vi "mkGetROIs.vi"(10 "Camera settings":T1={"Gain [1-4]"=0.0, "Offset"=0, "Mode"=0, "ROIs"=[], "ROI Size"={"X"=0, "Y"=0}, "Number of buffers"=40, "Use hardware multiple-ROI?"=TRUE, "GenericCameraConfig"={"Framerate (Hz)"=60, "Exposure time (us)"=5000, "Image size"={"Width"=1280, "Height"=1024}, "Number of buffers"=30}}, 11 "IMAQ Refnum in":refnum<k11>) -> (2 "Camera settings (out)":T1={"Gain [1-4]"=0.0, "Offset"=0, "Mode"=0, "ROIs"=[], "ROI Size"={"X"=0, "Y"=0}, "Number of buffers"=40, "Use hardware multiple-ROI?"=TRUE, "GenericCameraConfig"={"Framerate (Hz)"=60, "Exposure time (us)"=5000, "Image size"={"Width"=1280, "Height"=1024}, "Number of buffers"=30}}, 3 "IMAQ Refnum out":refnum<k11>)   [LabVIEW 2011]
uses:
  CameraConfig.ctl
  Main/Camera/GenericCameraConfigType.ctl
panel:
  out "#ROI":i32
  # "us"
  # "us"
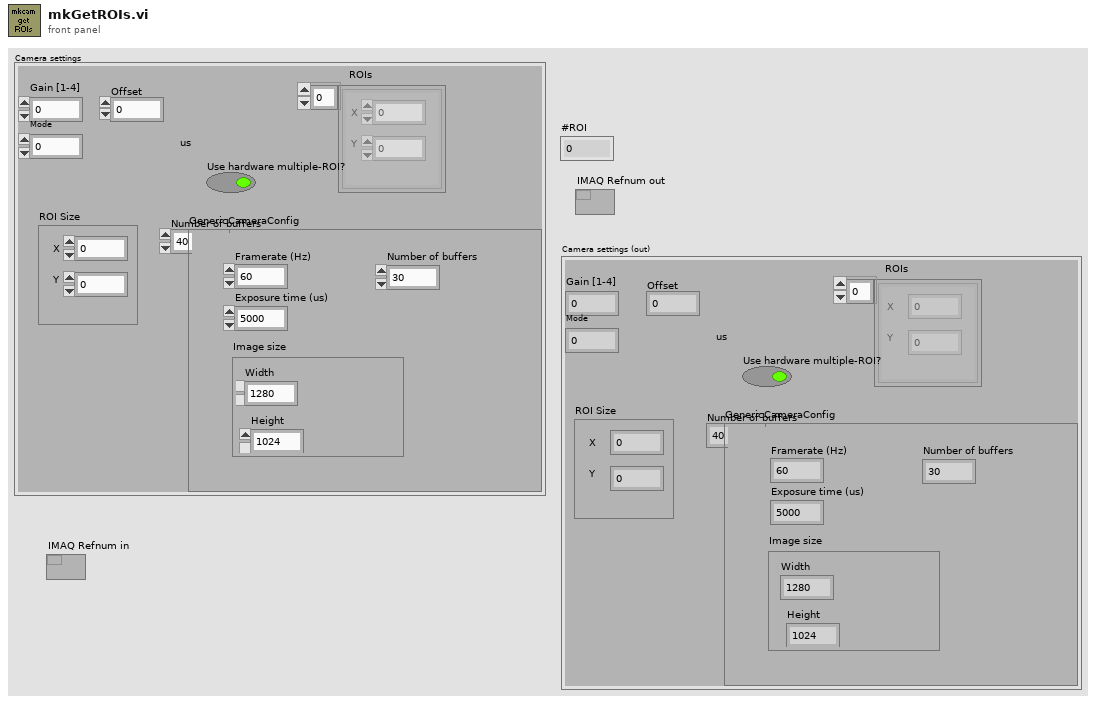
[diagram p1: front panel]
types:
  T1 = typedef "CameraConfig.ctl" = cluster{"Gain [1-4]":sgl, "Offset":i16, "Mode":i16, "ROIs":cluster{"X":i32, "Y":i32}[], "ROI Size":cluster{"X":i32, "Y":i32}, "Number of buffers":i32, "Use hardware multiple-ROI?":bool, "GenericCameraConfig":T2}
  T2 = typedef "GenericCameraConfigType.ctl" = cluster{"Framerate (Hz)":i32, "Exposure time (us)":i32, "Image size":cluster{"Width":i32, "Height":i32}, "Number of buffers":i32}
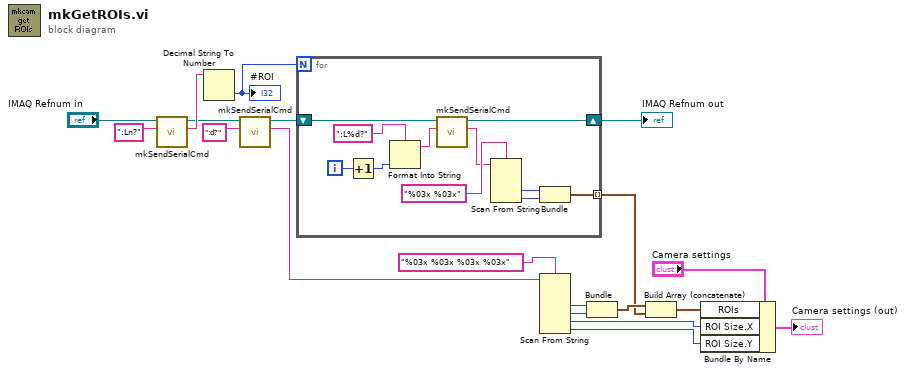
[diagram p0: block diagram]
diagram:
  n1 = call "mkSendSerialCmd.vi"("String"=":Ln?", "IMAQ Refnum in"="IMAQ Refnum in") -> ("String Read"=w17:string, "IMAQ Refnum out"=w16:refnum<k11>)  [unwired: 6 in, 2 out]
  n2 = Decimal String To Number(string=w17) -> (number=w4:i32)  [unwired: 2 in, 1 out]
  "#ROI" <- w4
  n3 = call "mkSendSerialCmd.vi"("String"=":d?", "IMAQ Refnum in"=w16) -> ("String Read"=w13:string, "IMAQ Refnum out"=w3:refnum<k11>)  [unwired: 6 in, 2 out]
  n4 = for {
    N: w4 -> [_]
    shift-right: [w29] -> w1
    shift-left: w3 -> [w30]
    tunnel: [w27] -> w2 mode=indexing
    i -> [w22]
    n5 = Increment(x=w22) -> (x+1=w21:i32)
    n6 = Format Into String(format string=":L%d?", w21) -> (resulting string=w20:string)  [unwired: 2 in, 1 out]
    n7 = call "mkSendSerialCmd.vi"("String"=w20, "IMAQ Refnum in"=w30) -> ("String Read"=w25:string, "IMAQ Refnum out"=w29:refnum<k11>)  [unwired: 6 in, 2 out]
    n8 = Scan From String(format string="%03x %03x", input string=w25) -> (output 1=w24:i32, output 2=w23:i32)  [unwired: 4 in, 3 out]
    n9 = Bundle(w24, w23) -> (w27:cluster{i32, i32})  [unwired: 1 in]
  }
  "IMAQ Refnum out" <- w1
  n10 = Scan From String(format string="%03x %03x %03x %03x", input string=w13) -> (output 1=w8:i32, output 2=w7:i32, output 3=w10:i32, output 4=w9:i32)  [unwired: 6 in, 3 out]
  n11 = Bundle(w8, w7) -> (w6:cluster{i32, i32})  [unwired: 1 in]
  n12 = Build Array (concatenate)(w6, w2) -> (w5:cluster{i32, i32}[])
  n13 = Bundle By Name(cluster="Camera settings", "ROIs"=w5, "ROI Size.X"=w10, "ROI Size.Y"=w9) -> (→"Camera settings (out)":T1)
